vi "Send.vi"(6 "Websocket Client Handler MTQ":refnum<class "Message Transport Queue.lvclass">, 7 "Message Priority":T1, 8 "error in (no error)":errorcluster, 9 "IP Address":string, 10 "GUID":string, 11 "Message Transport Queue":refnum<class "Message Transport Queue.lvclass">) -> (0 "error out":errorcluster)   [LabVIEW 2016, in "WebSocket Networking.lvlib" / "Add Connected Client to WSserver Msg.lvclass"]
doc: "--\nCopyright © 2017 Composed SystemsI All rights reserved.\n\nAuthor: Jon McBee <jon.mcbee@composed.io>\n\nThis library is provided \"AS IS\" ,WITHOUT WARRANTIES OR\nCONDITIONS OF ANY KIND, either express or implied.\n\nComposed Systems -- composed.io\n\nStream 0.0.1.1\nJon McBee - Composed Systems\nCopyright (c) 2017, Composed Systems"
uses:
  <userlib>/Common Components/WebSocket Networking/WS Server Msgs/Add Connected Client to WSserver Msg/Add Connected Client to WSserver Msg.lvclass
  <userlib>/Composed Systems/Stream/Mediator/Classes/Message Transport Queue/Message Transport Queue.lvclass
  <userlib>/Composed Systems/Stream/Mediator/Classes/Message Transport Interface/Message Priority.ctl
  C:/Program Files (x86)/National Instruments/LabVIEW 2016/user.lib/Composed Systems/Stream/Mediator/Classes/Message Interface/Message Interface.lvclass
  <userlib>/Common Components/WebSocket Networking/WS Server Msgs/Add Connected Client to WSserver Msg/Add Connected Client to WSserver Msg.lvclass/Add Connected Client to WSserver Msg.ctl
  <userlib>/Composed Systems/Stream/Mediator/Classes/Message Transport Interface/Message Transport Interface.lvclass
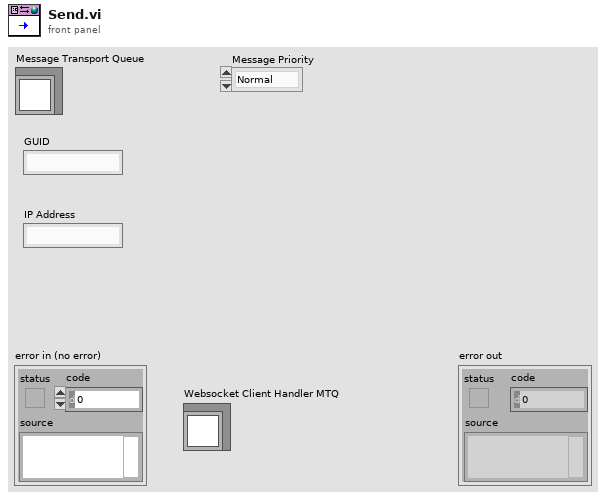
[diagram p1: front panel]
types:
  T1 = typedef "Stream Mediator.lvlib/Message Transport Interface.lvclass/Message Priority.ctl" = enum16{"Normal", "High"}
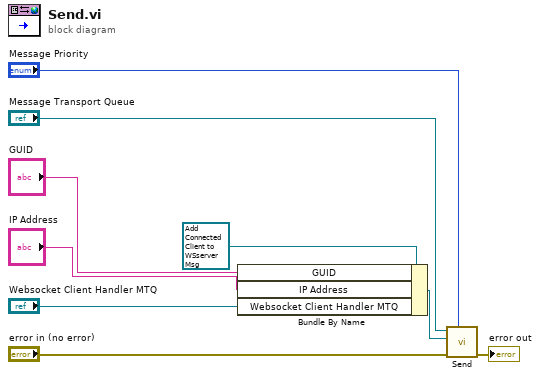
[diagram p0: block diagram]
diagram:
  n1 = Bundle By Name(cluster=refnum<class "Add Connected Client to WSserver Msg.lvclass"> refnum ("Stream Mediator.lvlib:Add Connected Client to WSserver Msg.lvclass"), "GUID"="GUID", "IP Address"="IP Address", "Websocket Client Handler MTQ"="Websocket Client Handler MTQ") -> (w6:refnum<class "Add Connected Client to WSserver Msg.lvclass">)
  n2 = call-dynamic "Send.vi"("Message Priority"="Message Priority", "error in (no error)"="error in (no error)", "Message"=w6, "Message Transport Queue in"="Message Transport Queue") -> ("error out"=→"error out":errorcluster)  [unwired: 5 in, 2 out]
